vi "1.4.2-Encoder Integration Simple.vi"(0 "Encoder B":bool, 5 "Encoder A":bool, 9 "Encoder A Old":bool, 11 "Encoder B Old":bool, 13 "Encoder Index":bool) -> (3 "Count Delta":i32, 4 "The Encoder Changed":bool, 6 "Count Zeroed at Index":i32, 8 "Encoder A Old (sReg)":bool, 10 "Encoder B Old (sReg)":bool)   [LabVIEW 2010]
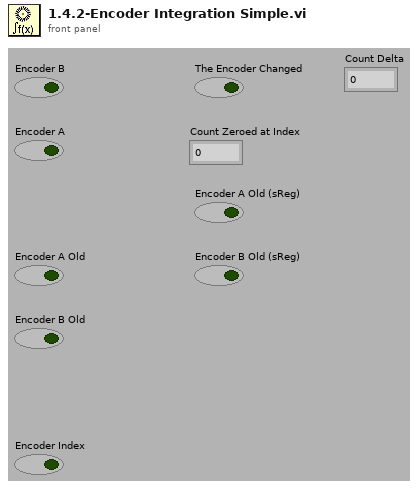
[diagram p1: front panel]
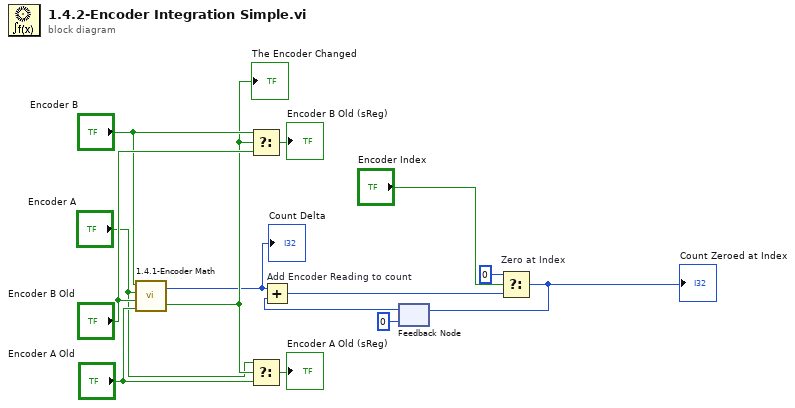
[diagram p0: block diagram]
diagram:
  n1 = call "1.4.1-Encoder Math.vi"("Encoder A_old"="Encoder A Old", "Encoder B_old"="Encoder B Old", "Encoder A_new"="Encoder A", "Encoder B_new"="Encoder B") -> ("The Encoder Changed"=w11:bool, "Change in Encoder Value"=w1:i32)
  "The Encoder Changed" <- w11
  "Count Delta" <- w1
  n2 = Select(t="Encoder B", s=w11, f="Encoder B Old") -> (s? t:f=→"Encoder B Old (sReg)":bool)
  n3 = Select(t="Encoder A", s=w11, f="Encoder A Old") -> (s? t:f=→"Encoder A Old (sReg)":bool)
  n4 = feedback #1(0) -> (w5:i32)
  n5 = Add "Add Encoder Reading to count"(x=w1, y=w5) -> (x+y=w2:i32)
  n6 = Select "Zero at Index"(t=0 ("Zero at Index"), s="Encoder Index", f=w2) -> (s? t:f=w3:i32)
  "Count Zeroed at Index" <- w3
  n7 = feedback-in #1(w3) -> ()
